vi "Export dat - LDLTS.vi"(8 "Error In":errorcluster, 9 "Workspace":path, 11 "LDLTS measurement":T1={"Name"="", "Comment"="", "Time"=timestamp(0 s since 1904-01-01), "Folder"=path "", "LDLTS properties"={"T"=0.0, "Test signal"=0.0, "Test frequency"=0.0, "Bandwidth"=0.0, "Averaging"=0.0, "Vbias"=0.0, "Vpulse"=0.0, "pulse length"=0.0, "Pulse 2"=FALSE, "Vpulse 2"=0.0, "pulse length 2"=0.0, "I range"=-2.0, "V range"=10.0, "Sampling rate"=0.0, "Acq. delay"=0.0, "Sampling time"=0.0}, "GUID"=""} {"LDLTS properties"."V range" items=["10mV"=0.01, "100mV"=0.1, "1V"=1.0, "10V"=10.0]; "LDLTS properties"."I range" items=["100nA"=-7.0, "1µA"=-6.0, "10µA"=-5.0, "100µA"=-4.0, "1mA"=-3.0, "10mA"=-2.0]}) -> (0 "Error Out":errorcluster)   [LabVIEW 2019]
doc: "Handles export of a LDLTS measurement to a .dat file, displays a GUI window"
uses:
  Type defs/LDLTS measurement Type Def.ctl
  Type defs/LDLTS properties Type Def.ctl
  <vilib>/Utility/sysdir.llb/System Directory Type.ctl
  <vilib>/Utility/file.llb/Write Delimited Spreadsheet (string).vi
  <vilib>/Utility/file.llb/Write Delimited Spreadsheet (DBL).vi
panel:
  out "String":string
  in  "Path":path caption="Export file as:"
  in  "Export":bool
  in  "Cancel":bool
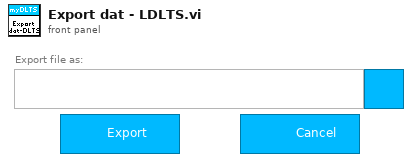
[diagram p1: front panel]
types:
  T1 = typedef "LDLTS measurement Type Def.ctl" = cluster{"Name":string, "Comment":string, "Time":timestamp, "Folder":path, "LDLTS properties":T2, "GUID":string}
  T2 = typedef "LDLTS properties Type Def.ctl" = cluster{"T":dbl[unit], "Test signal":dbl[unit], "Test frequency":dbl[unit], "Bandwidth":dbl[unit], "Averaging":dbl, "Vbias":dbl[unit], "Vpulse":dbl[unit], "pulse length":dbl[unit], "Pulse 2":bool, "Vpulse 2":dbl[unit], "pulse length 2":dbl[unit], "I range":dbl, "V range":dbl[unit], "Sampling rate":dbl[unit], "Acq. delay":dbl[unit], "Sampling time":dbl[unit]}
  T3 = enum32{"existing file", "new file", "new or existing file", "existing dir", "new dir", "new or existing dir", "existing file (use LLBs)", "new file (use LLBs)", "new or existing file (use LLBs)", "new or existing file or directory (use LLBs)", "existing dir (use LLBs)", "new dir (use LLBs)", "new or existing dir (use LLBs)", "existing file or dir", "new file or dir", "new or existing file or dir", "existing file or dir (use LLBs)", "new file or dir (use LLBs)"}
  T4 = typedef "System Directory Type.ctl" = i32
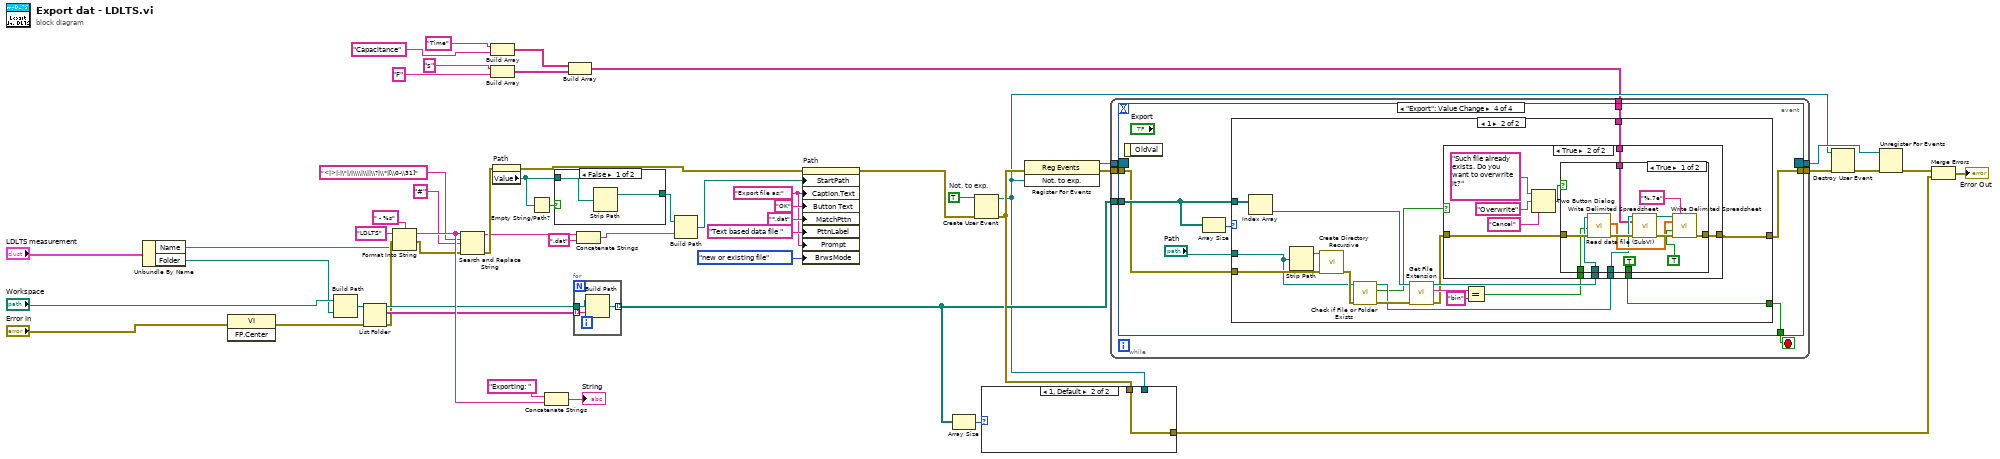
[diagram p0: block diagram]
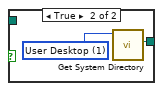
[diagram p2: hidden frame]
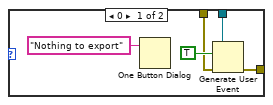
[diagram p3: hidden frame]
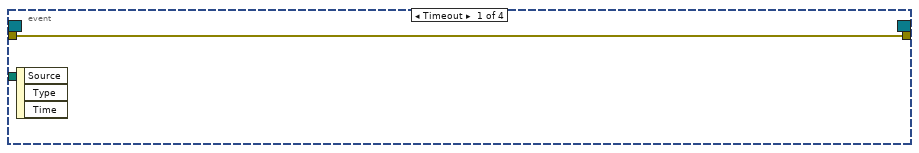
[diagram p4: hidden frame]
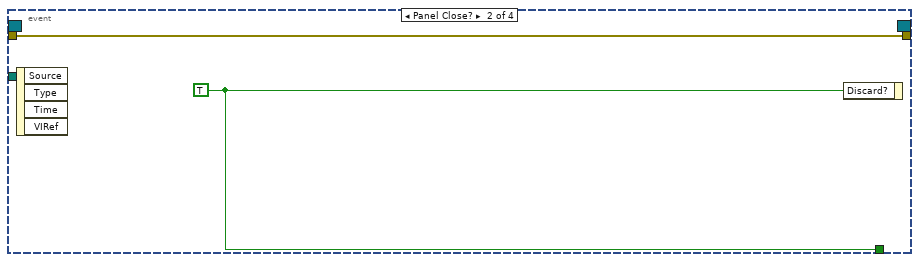
[diagram p5: hidden frame]
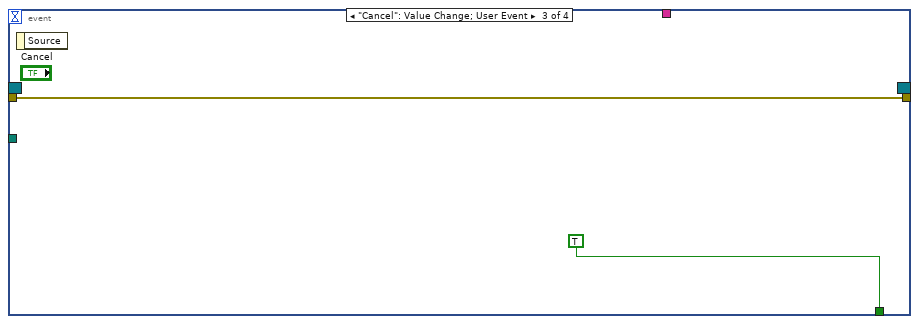
[diagram p6: hidden frame]
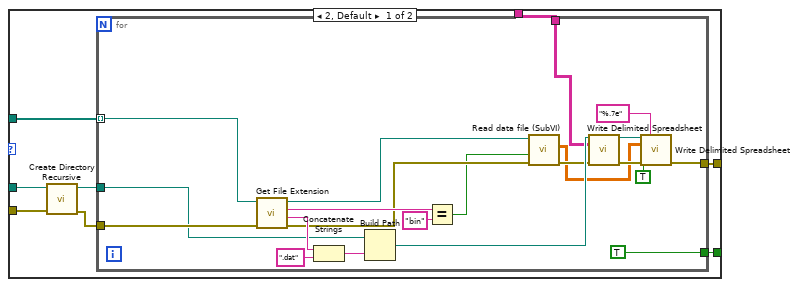
[diagram p7: hidden frame]
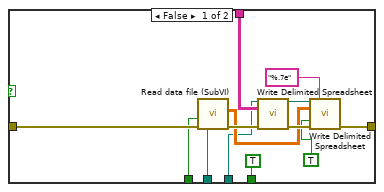
[diagram p8: hidden frame]
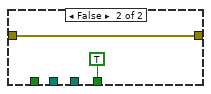
[diagram p9: hidden frame]
diagram:
  w22 = "Export file as:"
  w51 = TRUE  # Not. to exp.
  n1 = Unbundle By Name("LDLTS measurement") -> ("Name"=w13:string, "Folder"=w27:path)
  n2 = invoke class="VI" method="FP.Center"(error in="Error In") -> (error out=w9:errorcluster)  [unwired: 2 in, 2 out]
  n3 = Build Path(base path="Workspace", name or relative path=w27) -> (appended path=w20:path)
  n4 = List Folder(path=w20, error in=w9) -> (path out=w19:path, filenames=w26:string[], error out=w15:errorcluster)  [unwired: 2 in, 1 out]
  n5 = Format Into String(format string=" - %s", initial string="LDLTS", error in=w15, w13) -> (resulting string=w38:string, error out=w14:errorcluster)
  n6 = Search and Replace String(input string=w38, search string="<|>|:|\"|/|\\\\|\\||\\?|\\*|[\\0-\\31]", replace string="#" ("replace string (\"\")"), error in=w14) -> (result string=w12:string, error out=w16:errorcluster)  [unwired: 4 in, 2 out]
  n7 = Build Array("Time", "Capacitance") -> (w5:string[])
  n8 = Build Array("s", "F") -> (w6:string[])
  n9 = property on="Path" class="Path"(error in=w16) -> (error out=w28:errorcluster, "Value"=w34:path)  [unwired: 1 in, 1 out]
  n10 = Empty String/Path?(string/path=w34) -> (empty?=w35:bool)
  n11 = Concatenate Strings("Exporting: " ("string"), w38) -> (→"String":string)
  n12 = case shown="False" w35 {
    tunnel: w34 -> [w55 _]
    tunnel: [w54 w56] -> w30
    frame False {
      n13 = Strip Path(path=w55) -> (stripped path=w54:path)  [unwired: 1 out]
    }
    frame True {
      w57 = T4 1 items=["User Home"=0, "User Desktop"=1, "User Documents"=2, "User Application Data"=3, "User Preferences"=4, "User Temporary"=5, "Public Documents"=6, "Public Application Data"=7, "Public Preferences"=8, "Public Cache"=13, "System Core Libraries"=9, "System Installed Libraries"=10, "Application Files"=11, "Boot Volume Root"=12] ("system directory type")
      n14 = call <vilib>:"Get System Directory.vi"("system directory type"=w57) -> ("system directory"=w56:path)  [unwired: 10 in]
    }
  }
  n15 = Build Array(w5, w6) -> (w4:string[][])
  n16 = for {
    tunnel: w19 -> [w60]
    tunnel: [w59] -> w46 mode=indexing
    tunnel: w26 -> [w58] mode=indexing
    n17 = Build Path(base path=w60, name or relative path=w58) -> (appended path=w59:path)
  }
  n18 = Concatenate Strings(w12, ".dat" ("string")) -> (w17:string)
  n19 = Build Path(base path=w30, name or relative path=w17) -> (appended path=w29:path)
  n20 = property on="Path" class="Path"(error in=w28, "StartPath"=w29, "Caption.Text"=w22, "Button Text"="OK", "MatchPttn"="*.dat", "PttnLabel"="Text based data file ", "Prompt"=w22, "BrwsMode"=T3."new or existing file" ("Browse Options:Selection Mode")) -> (error out=w48:errorcluster)  [unwired: 1 in, 1 out]
  n21 = Array Size(array=w46) -> (size(s)=w52:i32)
  n22 = Create User Event(user event datatype=w51, error in=w48) -> (user event=w42:refnum<user-event>, error out=w47:errorcluster)
  n23 = case shown="1, Default" w52 {
    tunnel: w42 -> [w64 _]
    tunnel: w47 -> [w62 w66]
    tunnel: [w61 w66] -> w39
    frame 0 {
      n24 = One Button Dialog(message="Nothing to export") -> ()  [unwired: 1 in, 1 out]
      n25 = Generate User Event(user event=w64, event data cluster=TRUE ("event data"), error in=w62) -> (error out=w61:errorcluster)  [unwired: 1 in, 1 out]
    }
    frame 1, Default {
    }
  }
  n26 = register-events(error in=w47, w42) -> (reference out=w49:refnum<event-registration>, error out=w50:errorcluster)  [unwired: 1 in]
  n27 = while {
    tunnel: w50 -> [w73]
    tunnel: [w72] -> w45
    tunnel: w46 -> [w70]
    tunnel: w49 -> [w69]
    tunnel: [w68] -> w43
    tunnel: w4 -> [w67]
    stop <- w71 stop-if-true
    n28 = event shown="[3] \"Export\": Value Change" {
      selector: w69 -> [_ _ _ _]
      dyn-events: [_ _ _ _] -> w68
      timeout: _ -> [_ _ _ _]
      tunnel: w73 -> [w74 w75 w77 w80]
      tunnel: [w74 w75 w77 w85] -> w72
      tunnel: [_ w76 TRUE ("Discard?") w79] -> w71
      tunnel: w70 -> [_ _ _ w83]
      tunnel: w67 -> [_ _ _ w84]
      event Timeout {
        n29 = event-data() -> ()  [unwired: 1 in, 3 out]
      }
      event Panel Close? {
        w76 = TRUE ("Discard?")
        n30 = event-data() -> ()  [unwired: 1 in, 4 out]
        n31 = event-data("Discard?"=w76) -> ()  [unwired: 1 in, 1 out]
      }
      event "Cancel": Value Change; User Event {
        n32 = event-data() -> ()  [unwired: 1 in, 1 out]
      }
      event "Export": Value Change {
        n33 = event-data() -> ()  [unwired: 1 in, 1 out]
        n34 = Array Size(array=w83) -> (size(s)=w82:i32)
        n35 = case shown="1" w82 {
          tunnel: [w93 w122] -> w79
          tunnel: w80 -> [w90 w126]
          tunnel: w83 -> [w92 w125]
          tunnel: "Path" -> [w89 w123]
          tunnel: [w91 w115] -> w85
          tunnel: w84 -> [w86 w116]
          frame 2, Default {
            n36 = call <vilib>:"Create Directory Recursive.vi"("error in (no error)"=w90, "directory"=w89) -> ("error out"=w88:errorcluster, "directory copy"=w87:path)  [unwired: 3 in, 1 out]
            n37 = for {
              tunnel: [TRUE] -> w93
              tunnel: w92 -> [w111] mode=indexing
              tunnel: [w97] -> w91
              tunnel: w88 -> [w107]
              tunnel: w87 -> [w106]
              tunnel: w86 -> [w94]
              n38 = call <vilib>:"Get File Extension.vi"("error in (no error)"=w107, "file"=w111) -> ("error out"=w101:errorcluster, "filename without extension"=w109:string, "lowercase file extension"=w114:string, "dup file"=w102:path)  [unwired: 5 in, 1 out]
              n39 = Concatenate Strings(w109, ".dat" ("string")) -> (w110:string)
              n40 = Build Path(base path=w106, name or relative path=w110) -> (appended path=w99:path)
              n41 = Equal?(x=w114, y="bin") -> (x = y?=w100:bool)
              n42 = call "Read data file (SubVI).vi"("error in"=w101, "Binary"=w100, "file path in"=w102) -> ("error out"=w96:errorcluster, "2D data"=w95:dbl[][])  [unwired: 6 in, 1 out]
              n43 = call-poly <vilib>:"Write Delimited Spreadsheet.vi"("file path (dialog if empty)"=w99, "2D data"=w94, "error in (no error)"=w96) -> ("new file path (Not A Path if cancelled)"=w98:path, "error out"=w104:errorcluster)  [unwired: 11 in]
              n44 = call-poly <vilib>:"Write Delimited Spreadsheet.vi"("file path (dialog if empty)"=w98, "format (%.3f)"="%.7e", "2D data"=w95, "append to file? (new file:F)"=TRUE, "error in (no error)"=w104) -> ("error out"=w97:errorcluster)  [unwired: 9 in, 1 out]
            }
          }
          frame 1 {
            n45 = Index Array(array=w125) -> (element=w124:path)  [unwired: 1 in]
            n46 = Strip Path(path=w123) -> (stripped path=w128:path)  [unwired: 1 out]
            n47 = call <vilib>:"Create Directory Recursive.vi"("error in (no error)"=w126, "directory"=w128) -> ("error out"=w127:errorcluster)  [unwired: 3 in, 2 out]
            n48 = call <vilib>:"Check if File or Folder Exists.vi"("error in (no error)"=w127, "path"=w123) -> ("error out"=w129:errorcluster, "file or folder exists?"=w118:bool, "dup path"=w121:path)  [unwired: 7 in]
            n49 = call <vilib>:"Get File Extension.vi"("error in (no error)"=w129, "file"=w124) -> ("error out"=w117:errorcluster, "lowercase file extension"=w131:string, "dup file"=w120:path)  [unwired: 5 in, 2 out]
            n50 = Equal?(x=w131, y="bin") -> (x = y?=w119:bool)
            n51 = case shown="True" w118 {
              tunnel: [w137 w155] -> w115
              tunnel: [TRUE w154] -> w122
              tunnel: w117 -> [w135 w149]
              tunnel: w121 -> [w132 w148]
              tunnel: w120 -> [w133 w147]
              tunnel: w119 -> [w134 w146]
              tunnel: w116 -> [w136 w145]
              frame False {
                n52 = call "Read data file (SubVI).vi"("error in"=w135, "Binary"=w134, "file path in"=w133) -> ("error out"=w140:errorcluster, "2D data"=w139:dbl[][])  [unwired: 6 in, 1 out]
                n53 = call-poly <vilib>:"Write Delimited Spreadsheet.vi"("file path (dialog if empty)"=w132, "2D data"=w136, "error in (no error)"=w140) -> ("new file path (Not A Path if cancelled)"=w141:path, "error out"=w143:errorcluster)  [unwired: 11 in]
                n54 = call-poly <vilib>:"Write Delimited Spreadsheet.vi"("file path (dialog if empty)"=w141, "format (%.3f)"="%.7e", "2D data"=w139, "append to file? (new file:F)"=TRUE, "error in (no error)"=w143) -> ("error out"=w137:errorcluster)  [unwired: 9 in, 1 out]
              }
              frame True {
                n55 = Two Button Dialog(message="Such file already exists. Do you want to overwrite it?", 1:"Cancel" ("F button name (\"Cancel\")"), 2:"Overwrite" ("T button name (\"OK\")")) -> (T button?=w150:bool)
                n56 = case shown="True" w150 {
                  tunnel: [w161 w169] -> w155
                  tunnel: [TRUE TRUE] -> w154
                  tunnel: w149 -> [w162 w169]
                  tunnel: w148 -> [w160 _]
                  tunnel: w147 -> [w159 _]
                  tunnel: w146 -> [w158 _]
                  tunnel: w145 -> [w156 _]
                  frame True {
                    n57 = call "Read data file (SubVI).vi"("error in"=w162, "Binary"=w158, "file path in"=w159) -> ("error out"=w164:errorcluster, "2D data"=w163:dbl[][])  [unwired: 6 in, 1 out]
                    n58 = call-poly <vilib>:"Write Delimited Spreadsheet.vi"("file path (dialog if empty)"=w160, "2D data"=w156, "error in (no error)"=w164) -> ("new file path (Not A Path if cancelled)"=w165:path, "error out"=w167:errorcluster)  [unwired: 11 in]
                    n59 = call-poly <vilib>:"Write Delimited Spreadsheet.vi"("file path (dialog if empty)"=w165, "format (%.3f)"="%.7e", "2D data"=w163, "append to file? (new file:F)"=TRUE, "error in (no error)"=w167) -> ("error out"=w161:errorcluster)  [unwired: 9 in, 1 out]
                  }
                  frame False {
                  }
                }
              }
            }
          }
        }
      }
    }
  }
  n60 = Destroy User Event(user event=w42, error in=w45) -> (error out=w44:errorcluster)
  n61 = Unregister For Events(event registration refnum=w43, error in=w44) -> (error out=w41:errorcluster)
  n62 = Merge Errors(w41, w39) -> (→"Error Out":errorcluster)
